vi "1.1 Stop All Motors.vi"   [LabVIEW 2010]
uses:
  <vilib>/eio/EIONode/EIONode.xnode
  <vilib>/rvi/eio/nirviEIOImplementation/nirviEIOImplementation.xnode
  <vilib>/rvi/eio/common/nirviEmuClasses.ctl
  <vilib>/rvi/eio/common/nirviEmuTemplateMethod_noerrors.vi
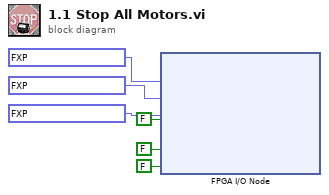
[diagram p0: block diagram]
diagram:
  n1 = xnode "FPGA I/O Node"("Steer Drive"=fxp<+/-,20,5> 0.0, "Lidar Drive"=fxp<+/-,20,5> 0.0, "Drive Motor"=fxp<+/-,20,5> 0.0, "Not E-Stopped"=FALSE ("Steer Drive Inhibit"), "Steering Motor Inhibit"=FALSE, "Lidar Motor Inhibit"=FALSE) -> ()  [unwired: 6 in, 6 out]
